vi "opposite enquece Keypad(SubVI).vi"(8 "error in (no error)":errorcluster, 9 "cmd":string, 10 "keypad cmd":string, 11 "Queue in":refnum<queue>) -> (0 "error out":errorcluster, 3 "Queue out":refnum<queue>)   [LabVIEW 2018]
uses:
  project/type defs/test keypad luster.ctl
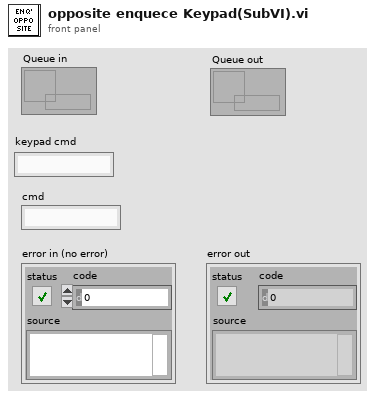
[diagram p1: front panel]
types:
  T1 = typedef "test keypad luster.ctl" = cluster{"cmd":string, "keypad cmd":variant}
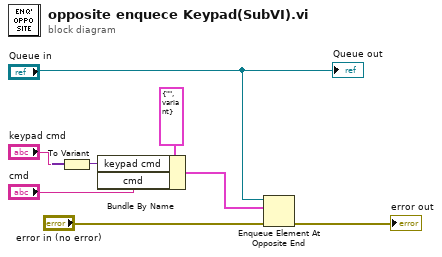
[diagram p0: block diagram]
diagram:
  n1 = To Variant(anything="keypad cmd") -> (Variant=w2:variant)
  n2 = Bundle By Name(cluster=T1 {"cmd"="", "keypad cmd"=variant(refnum<visa-resource-name> "")}, "keypad cmd"=w2, "cmd"="cmd") -> (w4:T1)
  n3 = Enqueue Element At Opposite End(queue="Queue in", element=w4, error in (no error)="error in (no error)") -> (error out=→"error out":errorcluster)  [unwired: 1 in, 2 out]
  "Queue out" <- "Queue in"
